vi "DoOperationStaticDispatchMethod Wrapper.vi"(8 "error in (no error)":errorcluster, 11 "SimpleArithmetic in":refnum<class "SimpleArithmetic.lvclass">) -> (0 "error out":errorcluster, 3 "SimpleArithmetic out":refnum<class "SimpleArithmetic.lvclass">)   [LabVIEW 2009]
uses:
  SimpleArithmetic.lvclass
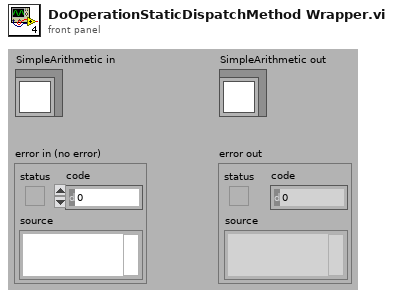
[diagram p1: front panel]
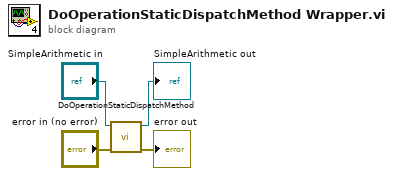
[diagram p0: block diagram]
diagram:
  n1 = call "DoOperationStaticDispatchMethod.vi"("error in (no error)"="error in (no error)", "SimpleArithmetic in"="SimpleArithmetic in") -> ("error out"=→"error out":errorcluster, "SimpleArithmetic out"=→"SimpleArithmetic out":refnum<class "SimpleArithmetic.lvclass">)  [unwired: 8 in]
